vi "Measurement.UI.SetControllerDependency.vi"(8 "error in (no error)":errorcluster, 10 "Measurement":refnum<class "Measurement.lvclass">, 11 "Measurement.WavelengthSweeping.UI in":refnum<class "Measurement.WavelengthSweeping.UI.lvclass">) -> (0 "error out":errorcluster, 3 "Measurement.WavelengthSweeping.UI out":refnum<class "Measurement.WavelengthSweeping.UI.lvclass">)   [LabVIEW 2019, in "Measurement.WavelengthSweeping.UI.lvclass"]
uses:
  Measurement.WavelengthSweeping.UI.lvclass
  Measurement/Measurement.lvclass
  Measurement.WavelengthSweeping/Measurement.WavelengthSweeping.lvclass
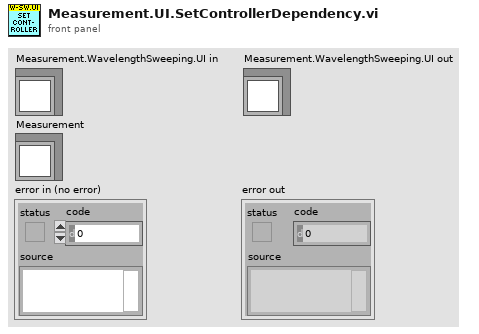
[diagram p1: front panel]
types:
  T1 = typedef "Measurement.WavelengthSweeping.UI.lvclass/Dependencies--Cluster.ctl" = cluster{"Measurement.WavelengthSweeping":refnum<class "Measurement.WavelengthSweeping.lvclass">}
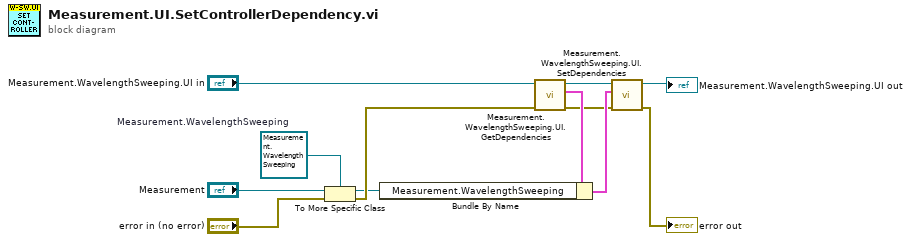
[diagram p0: block diagram]
diagram:
  w11 = refnum<class "Measurement.WavelengthSweeping.lvclass"> refnum  # Measurement.WavelengthSweeping
  n1 = To More Specific Class(target class=w11, reference="Measurement", error in="error in (no error)") -> (specific class reference=w6:refnum<class "Measurement.WavelengthSweeping.lvclass">, error out=w8:errorcluster)
  n2 = call "Measurement.WavelengthSweeping.UI.GetDependencies.vi"("error in (no error)"=w8, "Measurement.WavelengthSweeping.UI in"="Measurement.WavelengthSweeping.UI in") -> ("error out"=w4:errorcluster, "Dependencies"=w7:T1, "Measurement.WavelengthSweeping.UI out"=w3:refnum<class "Measurement.WavelengthSweeping.UI.lvclass">)  [unwired: 7 in]
  n3 = Bundle By Name(cluster=w7, "Measurement.WavelengthSweeping"=w6) -> (w5:T1)
  n4 = call "Measurement.WavelengthSweeping.UI.SetDependencies.vi"("error in (no error)"=w4, "Dependencies"=w5, "Measurement.WavelengthSweeping.UI in"=w3) -> ("error out"=→"error out":errorcluster, "Measurement.WavelengthSweeping.UI out"=→"Measurement.WavelengthSweeping.UI out":refnum<class "Measurement.WavelengthSweeping.UI.lvclass">)  [unwired: 7 in]
